vi "finishDirectKickPlay.vi"(8 "error in (no error)":errorcluster, 10 "Game":refnum<class "Game.lvclass">, 11 "DirectKickPlay in":refnum<class "DirectKickPlay.lvclass">) -> (0 "error out":errorcluster, 2 "result":bool, 3 "DirectKickPlay out":refnum<class "DirectKickPlay.lvclass">)   [LabVIEW 2021, in "DirectKickPlay.lvclass"]
uses:
  DirectKickPlay.lvclass
  Game_class/Game.lvclass
  Referee_class/command_interpreted.ctl
  Game_class/Game.lvclass/Game.ctl
  Events_class/Events.lvclass/Events.ctl
  Referee_class/Referee.lvclass/Referee.ctl
  Game_class/Read Referee.vi
  Referee_class/Read command_interpreted.vi
  Game_class/Read EventsRef.vi
  Events_class/Read ball_out.vi
  Events_class/Read kick.vi
  Events_class/Events.lvclass
  Referee_class/Referee.lvclass
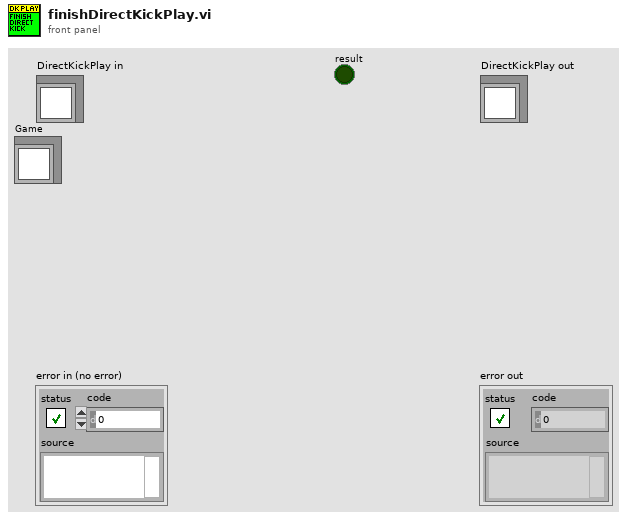
[diagram p1: front panel]
types:
  T1 = typedef "command_interpreted.ctl" = enum16{"Goal Ally", "Goal Enemy", "Ball Placement Enemy", "Ball Placement Ally", "Normal Half Time", "Extra Time  Break", "Extra Half Time", "None", "Post Game", "PKA Normal Start", "Prepare Kickoff Ally", "PKE Normal Start", "Prepare Kickoff Enemy", "Force Start", "Halt", "Timeout", "Prepare Penalty Ally", "Prepare Penalty Enemy", "PPA NormalStart", "PPE Normal Start", "Indirect Free Ally", "Direct Free Enemy", "Direct Free Ally", "Indirect Free Enemy", "Stop"}
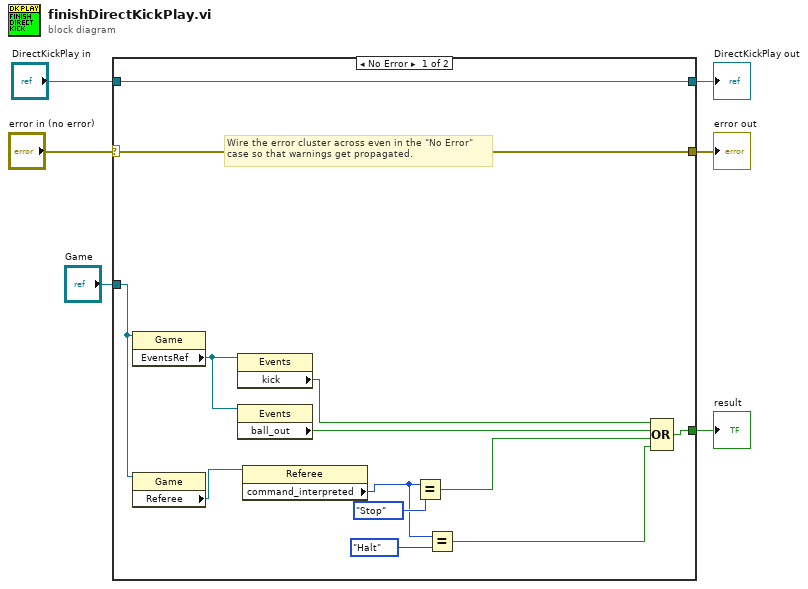
[diagram p0: block diagram]
diagram:
  n1 = case shown="No Error" "error in (no error)" {
    selector: "error in (no error)" -> [w18 w21]
    tunnel: [w18 w21] -> w5
    tunnel: [w19 w20] -> w3
    tunnel: "DirectKickPlay in" -> [w19 w20]
    tunnel: "Game" -> [w14 _]
    tunnel: [w13 _] -> w1
    frame No Error {
      # "Wire the error cluster across even in the \"No Error\"\ncase so that warnings get propagated."
      n2 = property class="Game"(reference=w14) -> ("EventsRef"=w15:refnum<class "Events.lvclass">)  [unwired: 1 in, 2 out]
      n3 = property class="Game"(reference=w14) -> ("Referee"=w17:refnum<class "Referee.lvclass">)  [unwired: 1 in, 2 out]
      n4 = property class="Events"(reference=w15) -> ("kick"=w7:bool)  [unwired: 1 in, 2 out]
      n5 = property class="Events"(reference=w15) -> ("ball_out"=w16:bool)  [unwired: 1 in, 2 out]
      n6 = property class="Referee"(reference=w17) -> ("command_interpreted"=w11:T1)  [unwired: 1 in, 2 out]
      n7 = Equal?(x=w11, y=command_interpreted."Stop") -> (x = y?=w9:bool)
      n8 = Equal?(x=w11, y=command_interpreted."Halt") -> (x = y?=w8:bool)
      n9 = Compound Arithmetic op=OR(w7, w16, w9, w8) -> (w13:bool)
    }
    frame Error {
    }
  }
  "error out" <- w5
  "DirectKickPlay out" <- w3
  "result" <- w1
